vi "BUILD_install for dependencies core.vi"(10 "LabVIEW Version":string, 11 "vipb path":path) -> (0 "error out":errorcluster)   [LabVIEW 2013]
uses:
  <vilib>/JKI/VIPM API/VIPM API_vipm_api.lvlib
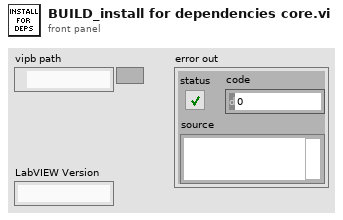
[diagram p1: front panel]
types:
  T1 = typedef "VIPM API_vipm_api.lvlib/Library Contents Cluster_vipm_api.ctl" = cluster{"Package Name":string, "Version":string, "Display Name":string, "Repository Name":string, "Company Name":string, "License Type":string, "Installed":bool, "Deprecated":bool, "Dependency or Conflict Problem":bool, "Downloaded":bool}
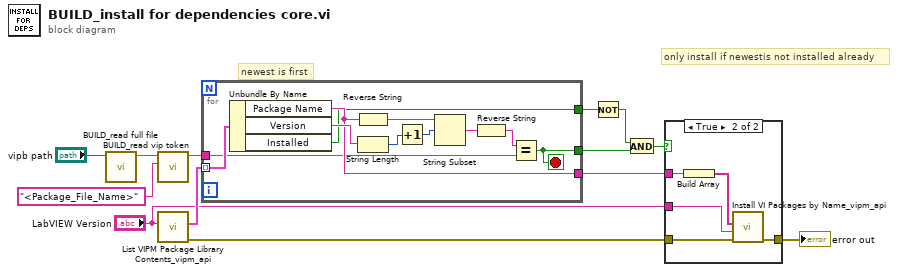
[diagram p0: block diagram]
diagram:
  # "only install if newestis not installed already"
  # "newest is first"
  n1 = call "BUILD_read full file.vi"("vip file"="vipb path") -> ("data"=w12:string)  [unwired: 9 in, 1 out]
  n2 = call "BUILD_read vip token.vi"("regular expression"="<Package_File_Name>", "data"=w12) -> ("trimmed string"=w11:string)  [unwired: 9 in]
  n3 = call <vilib>:"List VIPM Package Library Contents_vipm_api.vi"("LabVIEW Version"="LabVIEW Version") -> ("error out"=w8:errorcluster, "Library Contents []"=w7:T1[])  [unwired: 9 in]
  n4 = for {
    tunnel: w7 -> [w24] mode=indexing
    tunnel: [w18] -> w9
    tunnel: [w16] -> w10
    tunnel: w11 -> [w15]
    tunnel: [w14] -> w2
    stop <- w16 stop-if-true
    n5 = Unbundle By Name(w24) -> ("Package Name"=w18:string, "Version"=w23:string, "Installed"=w14:bool)
    n6 = Reverse String(1:w18) -> (0:w20:string)
    n7 = String Length(string=w23) -> (length=w22:i32)
    n8 = Increment(x=w22) -> (x+1=w21:i32)
    n9 = String Subset(string=w20, offset (0)=w21) -> (substring=w19:string)  [unwired: 1 in]
    n10 = Reverse String(1:w19) -> (0:w17:string)
    n11 = Equal?(x=w17, y=w15) -> (x = y?=w16:bool)
  }
  n12 = Not(x=w2) -> (.not. x?=w1:bool)
  n13 = And(x=w1, y=w10) -> (x .and. y?=w3:bool)
  n14 = case shown="True" w3 {
    tunnel: [w25 w26] -> w5
    tunnel: "LabVIEW Version" -> [_ w28]
    tunnel: w8 -> [w25 w27]
    tunnel: w9 -> [_ w30]
    frame False {
    }
    frame True {
      n15 = Build Array(w30) -> (w29:string[])
      n16 = call <vilib>:"Install VI Packages by Name_vipm_api.vi"("error in (no error)"=w27, "LabVIEW Version"=w28, "Package Names to Install []"=w29) -> ("error out"=w26:errorcluster)  [unwired: 8 in]
    }
  }
  "error out" <- w5
